vi "GetAllLibOrphanClass.vi"(6 "Get From All Src Folder?":bool, 7 "ListForChangedLibrariesOnly":bool, 8 "error in (no error)":errorcluster, 11 "Workspace Path":path) -> (0 "error out":errorcluster, 2 "Lib / Class Path []":path[](array[path]), 3 "Lib / Class Name []":string[](array[string]))   [LabVIEW 2019, in "Hawkeye.lvlib"]
uses:
  Hawkeye.lvlib
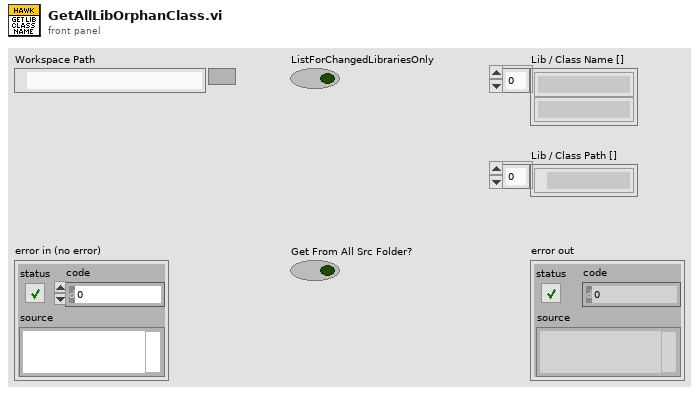
[diagram p1: front panel]
types:
  T1 = typedef "Hawkeye.lvlib/HawkeyePathConfigs.ctl" = cluster{"GlobalIncludePaths":path[], "GlobalExcludePaths":path[], "BuildSpecsIncludePaths":path[], "ActualDepsIncludePaths":path[], "WorkspacePath":path, "SourceFolderPaths":path[], "ChangedFilesLogpaths":map{string, path}}
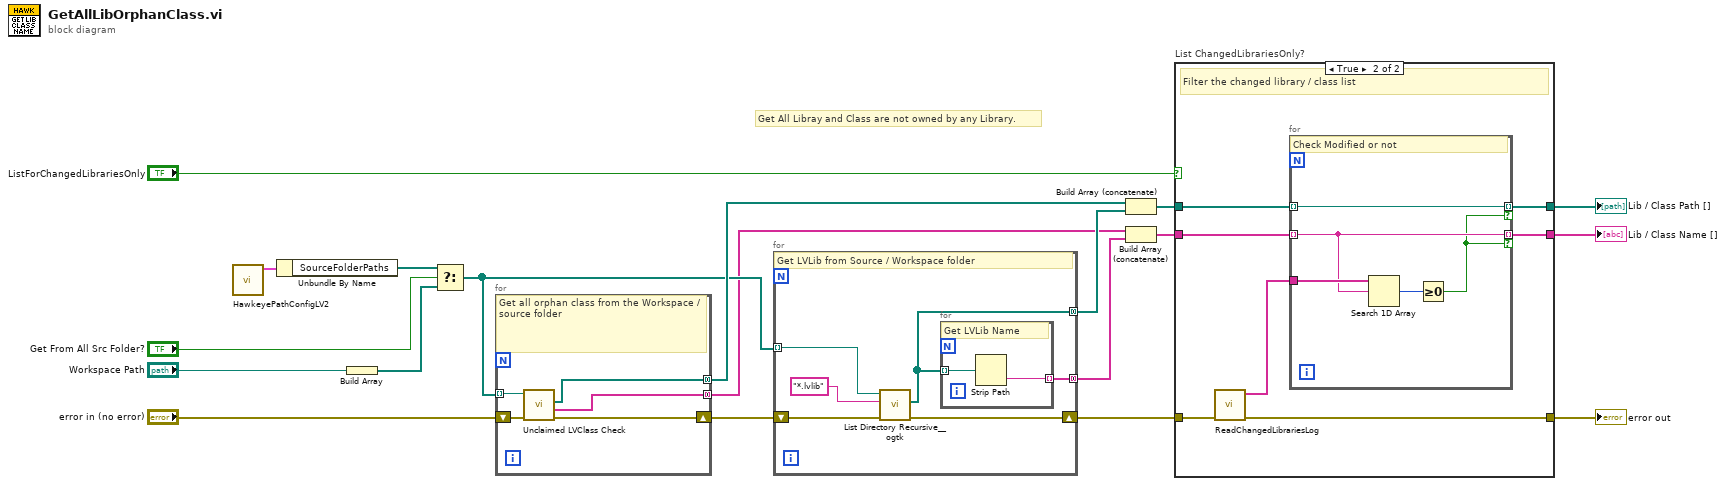
[diagram p0: block diagram]
diagram:
  # "Get All Libray and Class are not owned by any Library."
  n1 = call "HawkeyePathConfigLV2.vi"() -> ("Hawkeye Path Config Out"=w11:T1)  [unwired: 11 in]
  n2 = Unbundle By Name(w11) -> ("SourceFolderPaths"=w10:path[])
  n3 = Build Array("Workspace Path") -> (w9:path[])
  n4 = Select(t=w10, s="Get From All Src Folder?", f=w9) -> (s? t:f=w8:path[])
  n5 = for {
    shift-right: [w24] -> w13
    shift-left: "error in (no error)" -> [w21]
    tunnel: w8 -> [w23] mode=indexing
    tunnel: [w22] -> w12 mode=concatenating
    tunnel: [w20] -> w7 mode=concatenating
    # "Get all orphan class from the Workspace / source folder"
    n6 = call "Unclaimed LVClass Check.vi"("error in (no error)"=w21, "Source Folder Path"=w23) -> ("error out"=w24:errorcluster, "Orphan class name []"=w20:string[], "Orphan class path []"=w22:path[])  [unwired: 5 in, 2 out]
  }
  n7 = for {
    tunnel: [w26] -> w14 mode=concatenating
    shift-right: [w27] -> w5
    shift-left: w13 -> [w30]
    tunnel: w8 -> [w28] mode=indexing
    tunnel: [w25] -> w6 mode=concatenating
    # "Get LVLib from Source / Workspace folder"
    n8 = call <userlib>:"List Directory Recursive__ogtk.vi"("error in (no error)"=w30, "pattern"="*.lvlib", "Path"=w28) -> ("error out"=w27:errorcluster, "file paths"=w26:path[])  [unwired: 5 in, 2 out]
    n9 = for {
      tunnel: w26 -> [w32] mode=indexing
      tunnel: [w31] -> w25 mode=indexing
      # "Get LVLib Name"
      n10 = Strip Path(path=w32) -> (name=w31:string)  [unwired: 1 out]
    }
  }
  n11 = Build Array (concatenate)(w12, w14) -> (w4:path[])
  n12 = Build Array (concatenate)(w7, w6) -> (w3:string[])
  n13 = case "List ChangedLibrariesOnly?" shown="True" "ListForChangedLibrariesOnly" {
    tunnel: w5 -> [w33 w42]
    tunnel: [w33 w41] -> w17
    tunnel: [w35 w37] -> w1
    tunnel: w4 -> [w35 w40]
    tunnel: [w34 w36] -> w2
    tunnel: w3 -> [w34 w39]
    frame False {
    }
    frame True {
      # "Filter the changed library / class list"
      n14 = call "ReadChangedLibrariesLog.vi"("error in (no error)"=w42) -> ("error out"=w41:errorcluster, "ChangedLibraries"=w38:string[])  [unwired: 9 in]
      n15 = for {
        tunnel: w40 -> [w46] mode=indexing
        tunnel: w39 -> [w45] mode=indexing
        tunnel: w38 -> [w47]
        tunnel: [w46] -> w37 mode=indexing if=w43
        tunnel: [w45] -> w36 mode=indexing if=w43
        # "Check Modified or not"
        n16 = Search 1D Array(1D array=w47, element=w45) -> (index of element=w44:i32)  [unwired: 1 in]
        n17 = Greater Or Equal To 0?(x=w44) -> (x >= 0?=w43:bool)
      }
    }
  }
  "error out" <- w17
  "Lib / Class Name []" <- w2
  "Lib / Class Path []" <- w1
